vi "New Off Wire Message.vi"(2 "error in":errorcluster, 3 "JSON string":string) -> (0 "error out":errorcluster, 1 "Off Wire Message":T1)   [LabVIEW 2016]
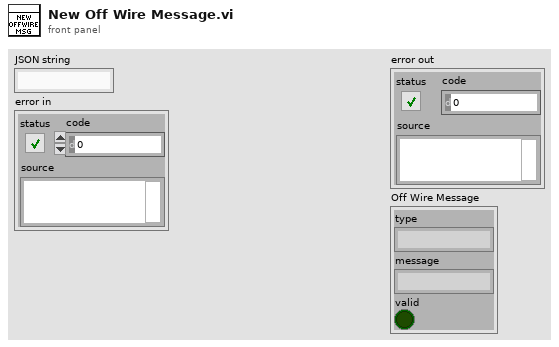
[diagram p1: front panel]
types:
  T1 = cluster{"type":string, "message":string, "valid":bool}
  T2 = cluster{"Type":string, "Message":string, "Valid":bool}
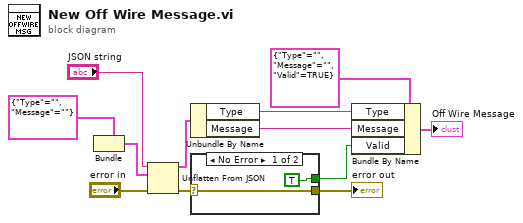
[diagram p0: block diagram]
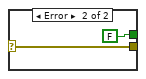
[diagram p2: hidden frame]
diagram:
  n1 = Bundle(cluster=cluster{"Type":string, "Message":string} {"Type"="", "Message"=""} ("input cluster")) -> (w10:cluster{"Type":string, "Message":string})  [unwired: 2 in]
  n2 = Unflatten From JSON(JSON string="JSON string", type and defaults=w10, error in (no error)="error in") -> (value=w9:cluster{"Type":string, "Message":string}, error out=w7:errorcluster)  [unwired: 4 in]
  n3 = Unbundle By Name(w9) -> ("Type"=w4:string, "Message"=w3:string)
  n4 = case shown="No Error" w7 {
    selector: w7 -> [w14 w16]
    tunnel: [w14 w16] -> w6
    tunnel: [TRUE FALSE] -> w2
    frame No Error {
    }
    frame Error {
    }
  }
  "error out" <- w6
  n5 = Bundle By Name(cluster=T2 {"Type"="", "Message"="", "Valid"=TRUE} ("input cluster"), "Type"=w4, "Message"=w3, "Valid"=w2) -> (→"Off Wire Message":T2)
